vi "MULTTCP_BlockingServer.vi"(1 "log":bool, 2 "logfile":path, 4 "cmdq":string, 5 "blockport":u16, 6 "cmdset":string, 7 "blockID":string, 8 "block notifier":refnum<notifier>, 10 "stot ref":refnum<vi>) -> ()   [LabVIEW 2016]
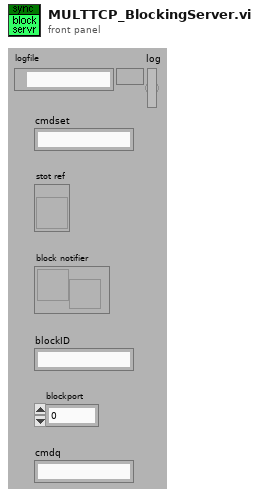
[diagram p1: front panel]
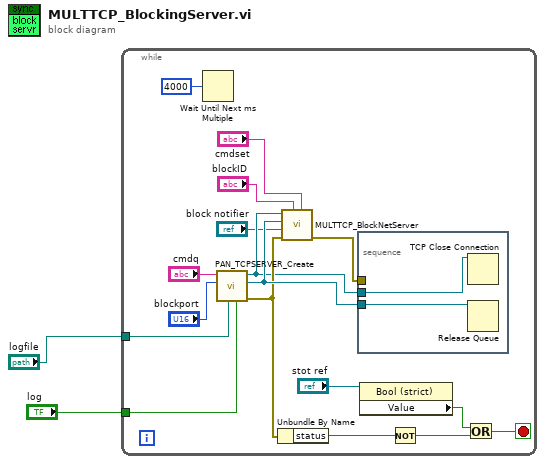
[diagram p0: block diagram]
diagram:
  n1 = while {
    tunnel: "logfile" -> [w4]
    tunnel: "log" -> [w3]
    stop <- w18 stop-if-true
    n2 = Wait Until Next ms Multiple(millisecond multiple=u32 4000) -> ()  [unwired: 1 out]
    n3 = call "PAN_TCPSERVER_Create.vi"("log"=w3, "logfile"=w4, "port"="blockport", "messages from socks Q name"="cmdq") -> ("error out"=w13:errorcluster, "queue out"=w14:refnum<queue>, "listener ID"=w11:refnum<k5>)  [unwired: 1 in, 4 out]
    n4 = Unbundle By Name(w13) -> ("status"=w15:bool)
    n5 = call "MULTTCP_BlockNetServer.vi"("cmdset"="cmdset", "ID"="blockID", "error in (no error)"=w13, "notifier In"="block notifier", "messages from sock"=w14, "listener ID"=w11) -> ("error out"=w12:errorcluster)  [unwired: 5 out]
    n6 = stacked-sequence {
      tunnel: w14 -> [w21]
      tunnel: w12 -> [_]
      tunnel: w11 -> [w20]
      frame #0 {
        n7 = TCP Close Connection(connection ID=w20) -> ()  [unwired: 1 in, 3 out]
        n8 = Release Queue(queue=w21) -> ()  [unwired: 1 in, 4 out]
      }
    }
    n9 = property class="Bool (strict)"(reference="stot ref") -> ("Value"=w16:bool)  [unwired: 1 in, 2 out]
    n10 = Not(x=w15) -> (.not. x?=w17:bool)
    n11 = Or(x=w16, y=w17) -> (x .or. y?=w18:bool)
  }
